vi "TS Status.vi"(8 "error in":errorcluster, 9 "New Data?":bool, 11 "Test Stand in":refnum<class "Generic Test Stand.lvclass">) -> (0 "error out":errorcluster, 3 "Test Stand out":refnum<class "Generic Test Stand.lvclass">)   [LabVIEW 2019, in "Generic Test Stand.lvclass"]
uses:
  Generic Test Stand.lvclass
  Generic Test Stand.lvclass/Generic Test Stand.ctl
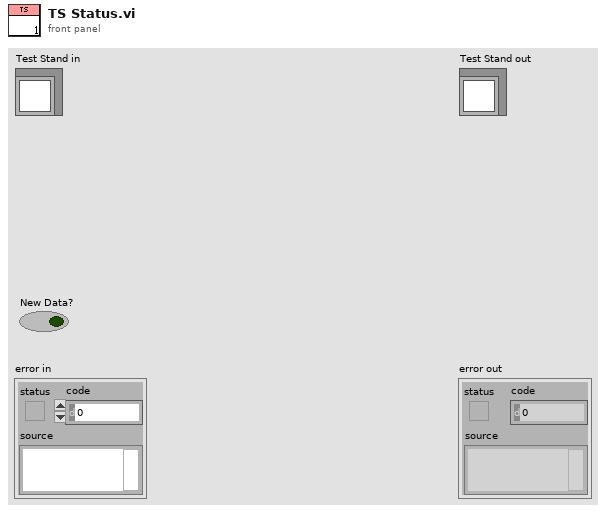
[diagram p1: front panel]
types:
  T1 = typedef "DAC Process.lvlib/DAC State.ctl" = enum16{"Idle", "Acquiring"}
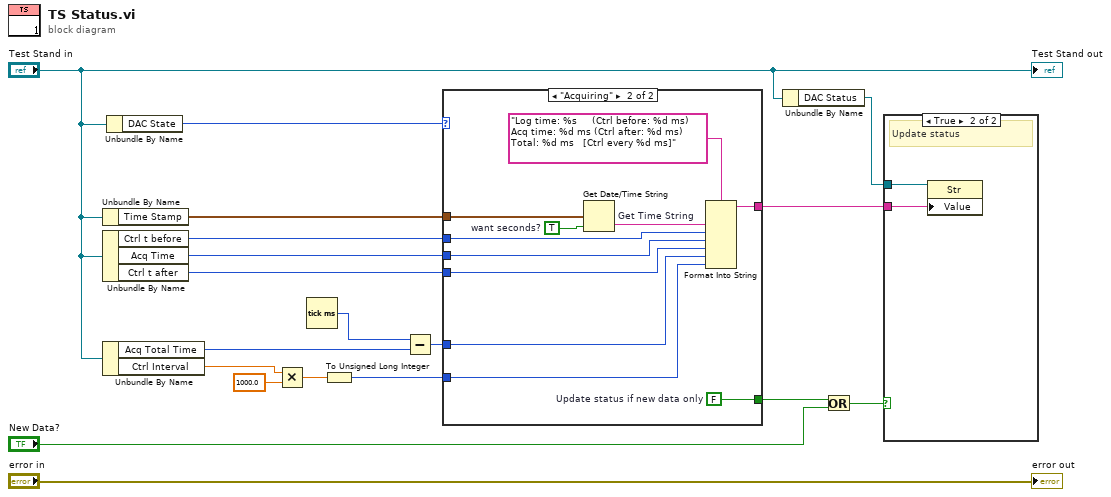
[diagram p0: block diagram]
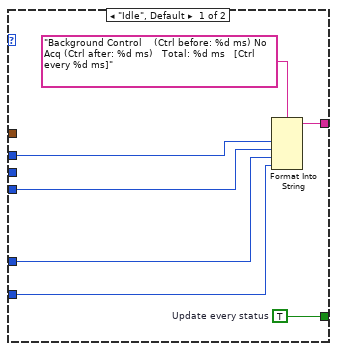
[diagram p3: hidden frame]
diagram:
  n1 = Unbundle By Name("Test Stand in") -> ("Time Stamp"=w10:timestamp)
  n2 = Unbundle By Name("Test Stand in") -> ("Ctrl t before"=w17:u32, "Acq Time"=w16:u32, "Ctrl t after"=w14:u32)
  n3 = Unbundle By Name("Test Stand in") -> ("Acq Total Time"=w15:u32, "Ctrl Interval"=w5:dbl)
  n4 = Unbundle By Name("Test Stand in") -> ("DAC State"=w11:T1)
  n5 = Multiply(x=w5, y=1000.0) -> (x*y=w7:dbl)
  n6 = Tick Count (ms)() -> (millisecond timer value=w8:u32)
  n7 = To Unsigned Long Integer(number=w7) -> (unsigned 32bit integer=w4:u32)
  n8 = Subtract(x=w8, y=w15) -> (x-y=w13:u32)
  n9 = case shown="\"Acquiring\"" w11 {
    tunnel: [w25 w36] -> w19
    tunnel: w17 -> [w24 w35]
    tunnel: w16 -> [_ w34]
    tunnel: w14 -> [w23 w33]
    tunnel: w13 -> [w22 w32]
    tunnel: w10 -> [_ w30]
    tunnel: w4 -> [w21 w28]
    tunnel: [w20 w27] -> w2
    frame "Idle", Default {
      w20 = TRUE  # Update every status
      n10 = Format Into String(format string="Background Control    (Ctrl before: %d ms) No Acq (Ctrl after: %d ms)   Total: %d ms   [Ctrl every %d ms]", w24, w23, w22, w21) -> (resulting string=w25:string)  [unwired: 2 in, 1 out]
    }
    frame "Acquiring" {
      w27 = FALSE  # Update status if new data only
      w31 = TRUE  # want seconds?
      n11 = Get Date/Time String "Get Time String"(seconds (now)=w30, want seconds? (F)=w31) -> (time string=w29:string)  [unwired: 1 in, 1 out]
      n12 = Format Into String(format string="Log time: %s     (Ctrl before: %d ms) Acq time: %d ms (Ctrl after: %d ms)   Total: %d ms   [Ctrl every %d ms]", w29, w35, w34, w33, w32, w28) -> (resulting string=w36:string)  [unwired: 2 in, 1 out]
    }
  }
  n13 = Unbundle By Name("Test Stand in") -> ("DAC Status"=w18:refnum<vi>)
  n14 = Or(x=w2, y="New Data?") -> (x .or. y?=w1:bool)
  n15 = case shown="True" w1 {
    tunnel: w19 -> [_ w39]
    tunnel: w18 -> [_ w38]
    frame False {
      # "Leave status as it is"
    }
    frame True {
      # "Update status"
      n16 = property class="Str"(reference=w38, "Value"=w39) -> ()  [unwired: 1 in, 2 out]
    }
  }
  "error out" <- "error in"
  "Test Stand out" <- "Test Stand in"
